vi "x_unit_offset.vi"(0 "spectrum x unit (wavenr/cm)":T1) -> (14 "xUnit val":i32)   [LabVIEW 2010, in "OSA.lvclass"]
doc: "SubVI to a <B>Thorlabs_OSA_64</B> object.\n\n[GOOP 1.0]"
uses:
  OSA.lvclass
  typeDef/spectrum_x_unit.ctl
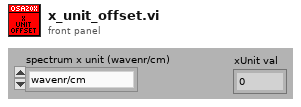
[diagram p1: front panel]
types:
  T1 = typedef "OSA.lvclass/spectrum_x_unit.ctl" = enum16{"wavenr/cm", "THz", "eV", "nm_air", "nm_vac"}
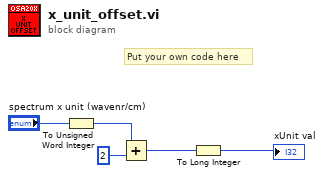
[diagram p0: block diagram]
diagram:
  # "Put your own code here"
  n1 = To Unsigned Word Integer(number="spectrum x unit (wavenr/cm)") -> (unsigned 16bit integer=w4:u16)
  n2 = Add(x=w4, y=u16 2) -> (x+y=w2:u16)
  n3 = To Long Integer(number=w2) -> (32bit integer=→"xUnit val":i32)
